vi "Read Numeric.vi"(8 "error in (no error)":errorcluster, 11 "Math in":refnum<class "Math.lvclass">) -> (0 "error out":errorcluster, 2 "Numeric":dbl, 3 "Math out":refnum<class "Math.lvclass">)   [LabVIEW 2016, in "Math.lvclass"]
uses:
  Math.lvclass
  Math.lvclass/Math.ctl
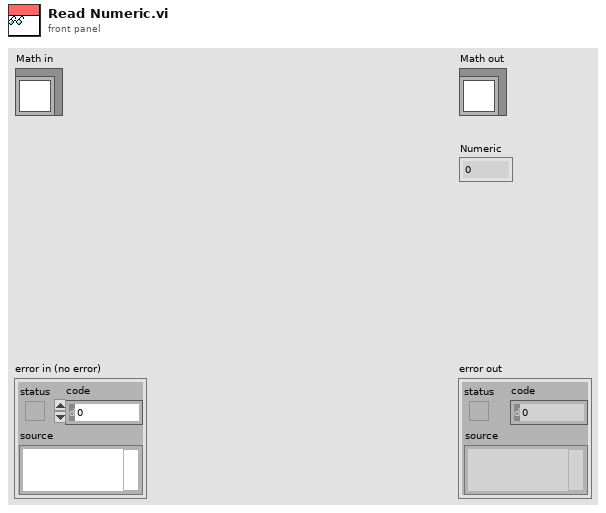
[diagram p1: front panel]
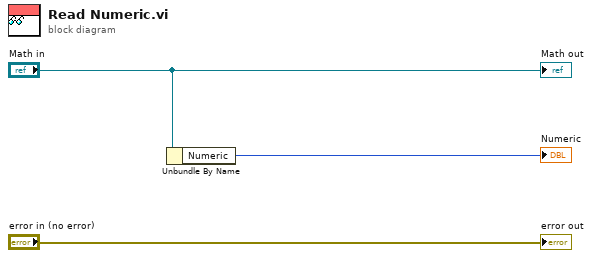
[diagram p0: block diagram]
diagram:
  n1 = Unbundle By Name("Math in") -> ("Numeric"=→"Numeric":i32)
  "error out" <- "error in (no error)"
  "Math out" <- "Math in"
